vi "Main.vi"(8 "Error In":errorcluster) -> (0 "Error Out":errorcluster)   [LabVIEW 2017, in "File IO.lvlib"]
uses:
  File IO.lvlib
  Controls/Params.ctl
  Controls/Commands [enum].ctl
  System Control/CTLs/Params.ctl
  DAQ/Controls/Params.ctl
  DAQ/Controls/DAQ Config.ctl
  DAQ/Controls/DAQ Indicators.ctl
  System Control/CTLs/Test Type.ctl
  Shutter Module/Controls/Params.ctl
  Monochromator/Controls/VISA parameters.ctl
  Monochromator/Controls/Params.ctl
  Monochromator/Controls/Type.ctl
  Monochromator/Controls/GratingValues.ctl
  Monochromator/Controls/Grating.ctl
  Monochromator/PTI/Controls/Params.ctl
  Monochromator/Custom Oriel drivers/Controls/Params.ctl
  C:/Project Work/icl-optical-software-rewrite/Optical Software Code Simplified/Modules/Monochromator/Cornerstone.dll
  Monochromator/Cornerstone.dll
  System Control/CTLs/Test params.ctl
  System Control/CTLs/Test Controls.ctl
  System Control/CTLs/Test indicators.ctl
  Scope/Controls/Params.ctl
  Scope/Controls/Models.ctl
  Scope/Controls/TPC.ctl
  Scope/Controls/Channels.ctl
  Trigger/Controls/Params.ctl
  Trigger/Controls/Mode.ctl
  Trigger/Controls/Trigger channels.ctl
  Scope/Controls/Acquisition type.ctl
  Scope/Controls/Record length.ctl
  Scope/Controls/Data.ctl
  Scope/Controls/Channel data.ctl
  Colour Wheel/Controls/Params.ctl
  Events/Controls/Action Refs [enum].ctl
  Controls/Config Cluster.ctl
  <userlib>/_OpenG.lib/file/file.llb/Valid Path - Traditional__ogtk.vi
  <vilib>/Utility/error.llb/Error Cluster From Error Code.vi
  <vilib>/ErrorRing/Error Ring.xnode
  System Control/Main controller.lvlib
  Events/Events.lvlib
  <vilib>/Utility/config.llb/NI_LVConfig.lvlib
  DAQ/DAQ.lvlib
  Serial comms/Serial comms.lvlib
  Shutter Module/Shutter.lvlib
  Monochromator/Monochromator.lvlib
  Monochromator/PTI/PTI.lvlib
  Monochromator/Custom Oriel drivers/Oriel (custom drivers).lvlib
  Scope/Scope.lvlib
  Trigger/Trigger.lvlib
  Colour Wheel/Colour Wheel.lvlib
  Processing/Processing.lvlib
panel:
  in  "Config":T1={"DAQ"={"Data"={"Live"={"t0"=timestamp(0 s since 1904-01-01), "dt"=1.0, "Y"=[]}, "Accumulated"={"t0"=timestamp(0 s since 1904-01-01), "dt"=1.0, "Y"=[]}, "Averaged"={"t0"=timestamp(0 s since 1904-01-01), "dt"=1.0, "Y"=[]}, "data array"=[], "live time array"=[], "Live (decimated)"={"t0"=timestamp(0 s since 1904-01-01), "dt"=1.0, "Y"=[]}}, "Config"={"Input Config"=10106, "Card"=enum."USB-6211", "100% Reflectance Standard (V)"=1.0, "Input Channel"="Dev2/ai0", "Average number of points"=50.0, "Trigger Level (V)"=0.4, "Rate (Hz)"=250000, "End Time (s)"=1.0}, "Indicators"={"Final number of points"=0.0, "Number of samples"=0.0, "dt"=0.0, "Shots"=1, "Shot counter"=0, "Test counter"=0, "Background level (V)"=0.0, "DAQ task"="", "timestamp of data"=timestamp(0 s since 1904-01-01), "Test Type"=enum."A-Test"}}, "Shutter"={"Open command string"="", "VISA"={"Timeout (ms)"=0, "Resource Name"="", "Baud Rate"=0, "Data Bits"=0, "Parity"=0, "Stop Bits"=0, "Flow Control"=0}}, "Monochromator"={"Type"=enum."Oriel", "Wavelength (nm)"=0.0, "Grating, gr/mm"=enum."2400", "Grating mode"=enum."Unknown", "Spectrum mode"={"Spectrum mode?"=FALSE, "Start wavelength (nm)"=0.0, "End wavelength (nm)"=0.0, "Wavelength step (nm)"=0.0, "Wavelength array"=[], "array index"=0}, "PTI"={"Delay before read (ms)"=0, "Mono 1"={"Timeout (ms)"=0, "Resource Name"="", "Baud Rate"=0, "Data Bits"=0, "Parity"=0, "Stop Bits"=0, "Flow Control"=0}, "Mono 2"={"Timeout (ms)"=0, "Resource Name"="", "Baud Rate"=0, "Data Bits"=0, "Parity"=0, "Stop Bits"=0, "Flow Control"=0}, "Two PTI Monochromators?"=FALSE}, "Oriel (custom)"={"reference"=refnum}, "Force wavelength confirmation (PTI)?"=FALSE}, "Test"={"Config"={"Amplification Factor"=0.0, "100% Reflectance Standard"=0.0, "Calculation Method"=enum."Reflectance", "Option to discard new data?"=FALSE, "Mode"=enum."Spectrum", "Number of Averages"=0, "B Test?"=FALSE}, "Indicators"={"DAQ Background Level (V)"=0.0, "A-Test Counter"=0, "B-Test Counter"=0, "Type"=enum."A-Test", "Scope Background Level (Amps)"=2.0, "TAS only?"=FALSE}}, "Scope"={"Config"={"VISA Resource"="USB0::0x0699::0x039D::C010764::INSTR", "Model"=enum."DPO 2012B", "Timebase"=0.0004, "Timeout (ms)"=60000, "TAS"={"Vertical Range (V)"=2.0, "Vertical Offset (0.0 divs)"=0.0, "Bandwidth"=0, "Probe Attenuation (10.0)"=1.0, "Vertical Coupling"=1, "Impedance"=0, "Multiplication factor"=1.0, "Channel"=enum."Channel 1"}, "TPC"={"Vertical Range (V)"=2.0, "Vertical Offset (0.0 divs)"=0.0, "Bandwidth"=0, "Probe Attenuation (10.0)"=1.0, "Vertical Coupling"=1, "Impedance"=0, "Multiplication factor"=1.0, "Channel"=enum."None"}, "Trigger"={"Mode"=enum."Laser (TAS)", "Source "=enum."Aux", "PIA"={"Test LEDs"=FALSE, "LED line"="", "LED off (s)"=0.0, "LED on (s)"=0.0}, "Threshold (V)"=0.8}}, "Indicators"={"Setup"={"Final number of points"=0.0, "Pretrigger points"=0.0, "Number of readouts"=0, "Model"={"Acquisition Type"=4, "Record length (points)"=1000, "Averages on scope"=4, "Average number of points"=10.0}}, "Timestamp of Data"=timestamp(0 s since 1904-01-01)}, "Data"={"TPC"={"Live data"={"t0"=timestamp(0 s since 1904-01-01), "dt"=1.0, "Y"=[]}, "Averaged data"={"t0"=timestamp(0 s since 1904-01-01), "dt"=1.0, "Y"=[]}, "Accumulated data"={"t0"=timestamp(0 s since 1904-01-01), "dt"=1.0, "Y"=[]}, "Final data"={"t0"=timestamp(0 s since 1904-01-01), "dt"=1.0, "Y"=[]}}, "TAS"={"Live data"={"t0"=timestamp(0 s since 1904-01-01), "dt"=1.0, "Y"=[]}, "Averaged data"={"t0"=timestamp(0 s since 1904-01-01), "dt"=1.0, "Y"=[]}, "Accumulated data"={"t0"=timestamp(0 s since 1904-01-01), "dt"=1.0, "Y"=[]}, "Final data"={"t0"=timestamp(0 s since 1904-01-01), "dt"=1.0, "Y"=[]}}, "Time arrays"={"Time array (decimated)"=[], "waveform"={"t0"=timestamp(0 s since 1904-01-01), "dt"=1.0, "Y"=[]}}}, "Test"={"Config"={"Amplification Factor"=0.0, "100% Reflectance Standard"=0.0, "Calculation Method"=enum."Reflectance", "Option to discard new data?"=FALSE, "Mode"=enum."Spectrum", "Number of Averages"=100, "B Test?"=FALSE}, "Indicators"={"DAQ Background Level (V)"=2.0, "A-Test Counter"=2, "B-Test Counter"=2, "Type"=enum."A-Test", "Scope Background Level (Amps)"=2.0, "TAS only?"=FALSE}}}, "Colour wheel"={"Reference"=0, "Colour Wheel Wavelengths"=[], "Waveform Index"=0, "COM Port"="", "Enabled?"=FALSE}, "File IO"={"Output Folder"=path "C:/Users/Abigail/Documents/Imperial Optical software/Optical Software Code Simplified/Output", "Error file"=path "C:/Users/Abigail/Documents/Imperial Optical software/Optical Software Code Simplified/Error Log.txt", "Config file"=path "C:/Users/Abigail/Documents/Imperial Optical software/Optical Software Code Simplified/Config.ini", "File prefix"="", "Waveform read"={"t0"=timestamp(0 s since 1904-01-01), "dt"=1.0, "Y"=[]}}} {"Scope"."Test"."Config"."Number of Averages" min=0; "Scope"."Indicators"."Setup"."Model"."Record length (points)" items=["1000"=1, "10,000"=10, "100,000"=100, "1,000,000"=1000, "5,000,000"=5000, "10,000,000"=10000]; "Scope"."Indicators"."Setup"."Model"."Acquisition Type" items=["Sample", "Peak Detect", "Hi Res", "Envelope", "Average"]; "Scope"."Config"."Trigger"."Threshold (V)" format="%#_3f"; "Scope"."Config"."TPC"."Impedance" items=["1M", "75", "50"]; "Scope"."Config"."TPC"."Vertical Coupling" items=["AC", "DC", "Ground"]; "Scope"."Config"."TPC"."Bandwidth" items=["FULL", "250 MHz", "150 MHz", "20 MHz"]; "Scope"."Config"."TAS"."Impedance" items=["1M", "75", "50"]; "Scope"."Config"."TAS"."Vertical Coupling" items=["AC", "DC", "Ground"]; "Scope"."Config"."TAS"."Bandwidth" items=["FULL", "250 MHz", "150 MHz", "20 MHz"]; "Scope"."Config"."Timebase" format="%^#_3e"; "Test"."Config"."Number of Averages" min=0; "Monochromator"."PTI"."Mono 2"."Flow Control" items=["1.0"=10, "1.5"=15, "2.0"=20]; "Monochromator"."PTI"."Mono 2"."Stop Bits" items=["None", "Odd", "Even", "Mark", "Space"]; "Monochromator"."PTI"."Mono 2"."Parity" items=["None", "Odd", "Even", "Mark", "Space"]; "Monochromator"."PTI"."Mono 1"."Flow Control" items=["1.0"=10, "1.5"=15, "2.0"=20]; "Monochromator"."PTI"."Mono 1"."Stop Bits" items=["None", "Odd", "Even", "Mark", "Space"]; "Monochromator"."PTI"."Mono 1"."Parity" items=["None", "Odd", "Even", "Mark", "Space"]; "Shutter"."VISA"."Flow Control" items=["None"=0, "XON/XOFF"=1, "RTS/CTS"=2, "DTR/DSR"=4]; "Shutter"."VISA"."Stop Bits" items=["1.0"=10, "1.5"=15, "2.0"=20]; "Shutter"."VISA"."Parity" items=["None", "Odd", "Even", "Mark", "Space"]; "DAQ"."Config"."Input Config" items=["default"=-1, "RSE"=10083, "NRSE"=10078, "Differential"=10106, "Pseudodifferential"=12529]}
  in  "State":T30
  in  "Stop Button":bool
  in  "Config":T29={"Output Folder"=path "C:/Users/Abigail/Documents/Imperial Optical software/Optical Software Code Simplified/Output", "Error file"=path "Error Log.txt", "Config file"=path "Config.ini", "File prefix"="600nm", "Waveform read"={"t0"=timestamp(0 s since 1904-01-01), "dt"=1.0, "Y"=[]}}
  out "Test":bool=TRUE
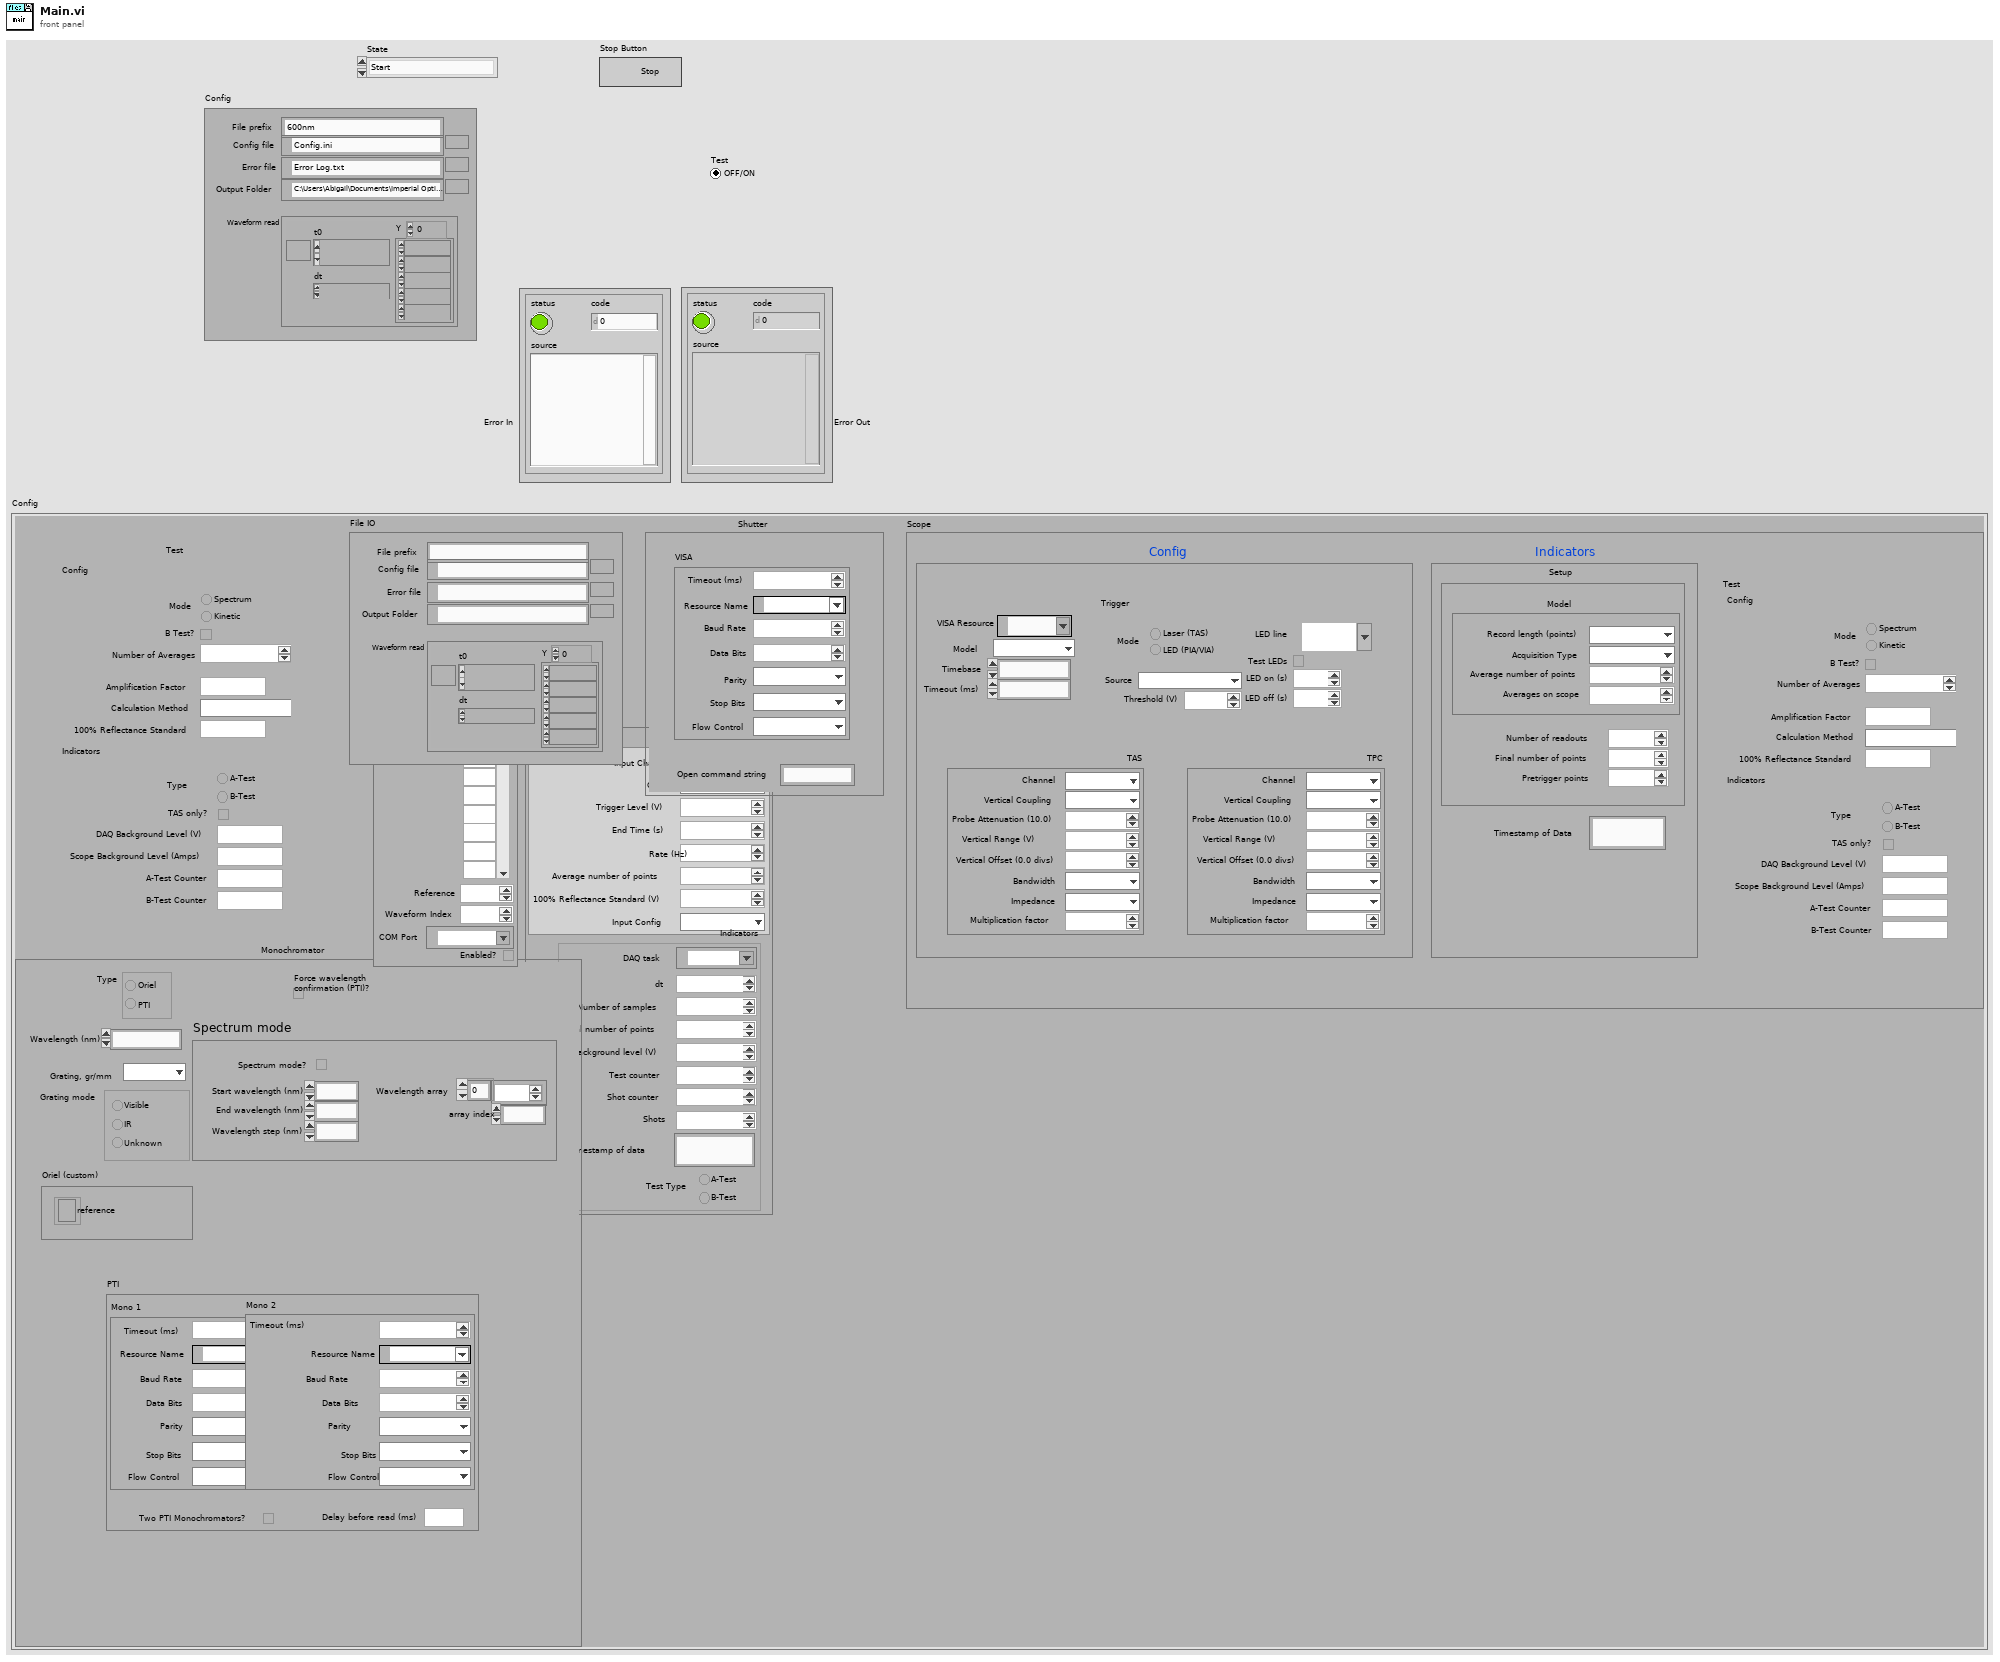
[diagram p1: front panel]
types:
  T1 = typedef "Main controller.lvlib/Params.ctl" = cluster{"DAQ":T2, "Shutter":T6, "Monochromator":T8, "Test":T14, "Scope":T17, "Colour wheel":T28, "File IO":T29}
  T2 = typedef "DAQ.lvlib/Params.ctl" = cluster{"Data":cluster{"Live":waveform(dbl), "Accumulated":waveform(dbl), "Averaged":waveform(dbl), "data array":dbl[], "live time array":dbl[], "Live (decimated)":waveform(dbl)}, "Config":T3, "Indicators":T4}
  T3 = typedef "DAQ.lvlib/DAQ Config.ctl" = cluster{"Input Config":i32, "Card":enum16{"USB-6211", "USB-6251", "USB-6361"}, "100% Reflectance Standard (V)":dbl, "Input Channel":tag, "Average number of points":dbl, "Trigger Level (V)":dbl, "Rate (Hz)":i32, "End Time (s)":dbl}
  T4 = typedef "DAQ.lvlib/DAQ Indicators.ctl" = cluster{"Final number of points":dbl, "Number of samples":dbl, "dt":dbl, "Shots":i32, "Shot counter":i32, "Test counter":i32, "Background level (V)":dbl, "DAQ task":refnum<k21>, "timestamp of data":timestamp, "Test Type":T5}
  T5 = typedef "Main controller.lvlib/Test Type.ctl" = enum32{"A-Test", "B-Test"}
  T6 = typedef "Shutter.lvlib/Params.ctl" = cluster{"Open command string":string, "VISA":T7}
  T7 = typedef "Serial comms.lvlib/VISA parameters.ctl" = cluster{"Timeout (ms)":u32, "Resource Name":refnum<visa-resource-name>, "Baud Rate":u32, "Data Bits":u16, "Parity":u16, "Stop Bits":u16, "Flow Control":u16}
  T8 = typedef "Monochromator.lvlib/Params.ctl" = cluster{"Type":T9, "Wavelength (nm)":dbl, "Grating, gr/mm":T10, "Grating mode":T11, "Spectrum mode":cluster{"Spectrum mode?":bool, "Start wavelength (nm)":dbl, "End wavelength (nm)":dbl, "Wavelength step (nm)":dbl, "Wavelength array":dbl[], "array index":u32}, "PTI":T12, "Oriel (custom)":T13, "Force wavelength confirmation (PTI)?":bool}
  T9 = typedef "Monochromator.lvlib/Type.ctl" = enum32{"Oriel", "PTI"}
  T10 = typedef "Monochromator.lvlib/GratingValues.ctl" = enum16{"2400", "1800", "1200", "600", "300", "150"}
  T11 = typedef "Monochromator.lvlib/Grating.ctl" = enum32{"Unknown", "Visible", "IR"}
  T12 = typedef "Monochromator.lvlib/PTI.lvlib/Params.ctl" = cluster{"Delay before read (ms)":u32, "Mono 1":T7, "Mono 2":T7, "Two PTI Monochromators?":bool}
  T13 = typedef "Monochromator.lvlib/Oriel (custom drivers).lvlib/Params.ctl" = cluster{"reference":refnum<k24>}
  T14 = typedef "Main controller.lvlib/Test params.ctl" = cluster{"Config":T15, "Indicators":T16}
  T15 = typedef "Main controller.lvlib/Test Controls.ctl" = cluster{"Amplification Factor":dbl, "100% Reflectance Standard":dbl, "Calculation Method":enum16{"Reflectance", "Transmission", "Kubelka-Munk"}, "Option to discard new data?":bool, "Mode":enum32{"Spectrum", "Kinetic"}, "Number of Averages":i32, "B Test?":bool}
  T16 = typedef "Main controller.lvlib/Test indicators.ctl" = cluster{"DAQ Background Level (V)":dbl, "A-Test Counter":i32, "B-Test Counter":i32, "Type":T5, "Scope Background Level (Amps)":dbl, "TAS only?":bool}
  T17 = typedef "Scope.lvlib/Params.ctl" = cluster{"Config":cluster{"VISA Resource":refnum<visa-resource-name>, "Model":T18, "Timebase":dbl, "Timeout (ms)":u32, "TAS":T19, "TPC":T19, "Trigger":T21}, "Indicators":cluster{"Setup":cluster{"Final number of points":dbl, "Pretrigger points":dbl, "Number of readouts":i32, "Model":cluster{"Acquisition Type":T24, "Record length (points)":T25, "Averages on scope":i32, "Average number of points":dbl}}, "Timestamp of Data":timestamp}, "Data":T26, "Test":T14}
  T18 = typedef "Scope.lvlib/Models.ctl" = enum16{"DPO 3012", "DPO 2012B", "TDS 3012C"}
  T19 = typedef "Scope.lvlib/TPC.ctl" = cluster{"Vertical Range (V)":dbl, "Vertical Offset (0.0 divs)":dbl, "Bandwidth":i32, "Probe Attenuation (10.0)":dbl, "Vertical Coupling":u16, "Impedance":u16, "Multiplication factor":dbl, "Channel":T20}
  T20 = typedef "Scope.lvlib/Channels.ctl" = enum16{"Channel 1", "Channel 2", "Channel 3", "Channel 4", "Math", "Reference A", "Reference B", "Reference C", "Reference D", "B1", "B2", "None"}
  T21 = typedef "Scope.lvlib/Trigger.lvlib/Params.ctl" = cluster{"Mode":T22, "Source ":T23, "PIA":cluster{"Test LEDs":bool, "LED line":tag, "LED off (s)":dbl, "LED on (s)":dbl}, "Threshold (V)":dbl}
  T22 = typedef "Scope.lvlib/Trigger.lvlib/Mode.ctl" = enum32{"Laser (TAS)", "LED (PIA/VIA)"}
  T23 = typedef "Scope.lvlib/Trigger.lvlib/Trigger channels.ctl" = enum16{"Channel 1", "Channel 2", "Channel 3", "Channel 4", "AC Line", "Aux", "Digital Channel 0", "Digital Channel 1", "Digital Channel 2", "Digital Channel 3", "Digital Channel 4", "Digital Channel 5", "Digital Channel 6", "Digital Channel 7", "Digital Channel 8", "Digital Channel 9", "Digital Channel 10", "Digital Channel 11", "Digital Channel 12", "Digital Channel 13", "Digital Channel 14", "Digital Channel 15", "RF"}
  T24 = typedef "Scope.lvlib/Acquisition type.ctl" = u16
  T25 = typedef "Scope.lvlib/Record length.ctl" = u32
  T26 = typedef "Scope.lvlib/Data.ctl" = cluster{"TPC":T27, "TAS":T27, "Time arrays":cluster{"Time array (decimated)":dbl[], "waveform":waveform(dbl)}}
  T27 = typedef "Scope.lvlib/Channel data.ctl" = cluster{"Live data":waveform(dbl), "Averaged data":waveform(dbl), "Accumulated data":waveform(dbl), "Final data":waveform(dbl)}
  T28 = typedef "Colour Wheel.lvlib/Params.ctl" = cluster{"Reference":i32, "Colour Wheel Wavelengths":dbl[], "Waveform Index":i32, "COM Port":refnum<visa-resource-name>, "Enabled?":bool}
  T29 = typedef "File IO.lvlib/Params.ctl" = cluster{"Output Folder":path, "Error file":path, "Config file":path, "File prefix":string, "Waveform read":waveform(dbl)}
  T30 = typedef "File IO.lvlib/Commands [enum].ctl" = enum16{"Start", "Stop", "Read waveform", "Write waveform", "Delete waveform", "Log error", "Write config", "Read config", "Save parameters", "Send waveform to processing", "Update file prefix"}
  T31 = enum32{"Bad", "Idle", "Run top level", "Running"}
  T32 = typedef "Events.lvlib/Action Refs [enum].ctl" = enum16{"Init", "Ref", "Kill"}
  T33 = typedef "Events.lvlib/Refs [cluster].ctl" = cluster{"Exit":refnum<user-event>, "Controller":refnum<user-event>, "System Error":refnum<user-event>, "UI":refnum<user-event>, "Example Module":refnum<user-event>, "Shutter":refnum<user-event>, "Monochromator":refnum<user-event>, "DAQ":refnum<user-event>, "Scope":refnum<user-event>, "Processing":refnum<user-event>, "File IO":refnum<user-event>, "Colour wheel":refnum<user-event>}
  T34 = enum16{"open", "replace", "create", "open or create", "replace or create", "replace or create with confirmation"}
  T35 = cluster{"Waveform Data":dbl[][], "Waveform Name":string}
  T36 = cluster{"Debug Waveform Read":dbl[][], "Waveform name":string}
  T37 = typedef "File IO.lvlib/Config Cluster.ctl" = cluster{"Test.Config":T15, "File IO":T29, "DAQ.Config":T3, "Monochromator":T8, "Scope.Config":cluster{"VISA Resource":refnum<visa-resource-name>, "Model":T18, "Timebase":dbl, "Timeout (ms)":u32, "TAS":T19, "TPC":T19, "Trigger":T21}, "Colour Wheel":T28, "Shutter":T6, "Scope.Setup.Model":cluster{"Acquisition Type":T24, "Record length (points)":T25, "Averages on scope":i32, "Average number of points":dbl}}
  T38 = typedef "NI_LVConfig.lvlib/Config Data RefNum.ctl" = refnum<k1>
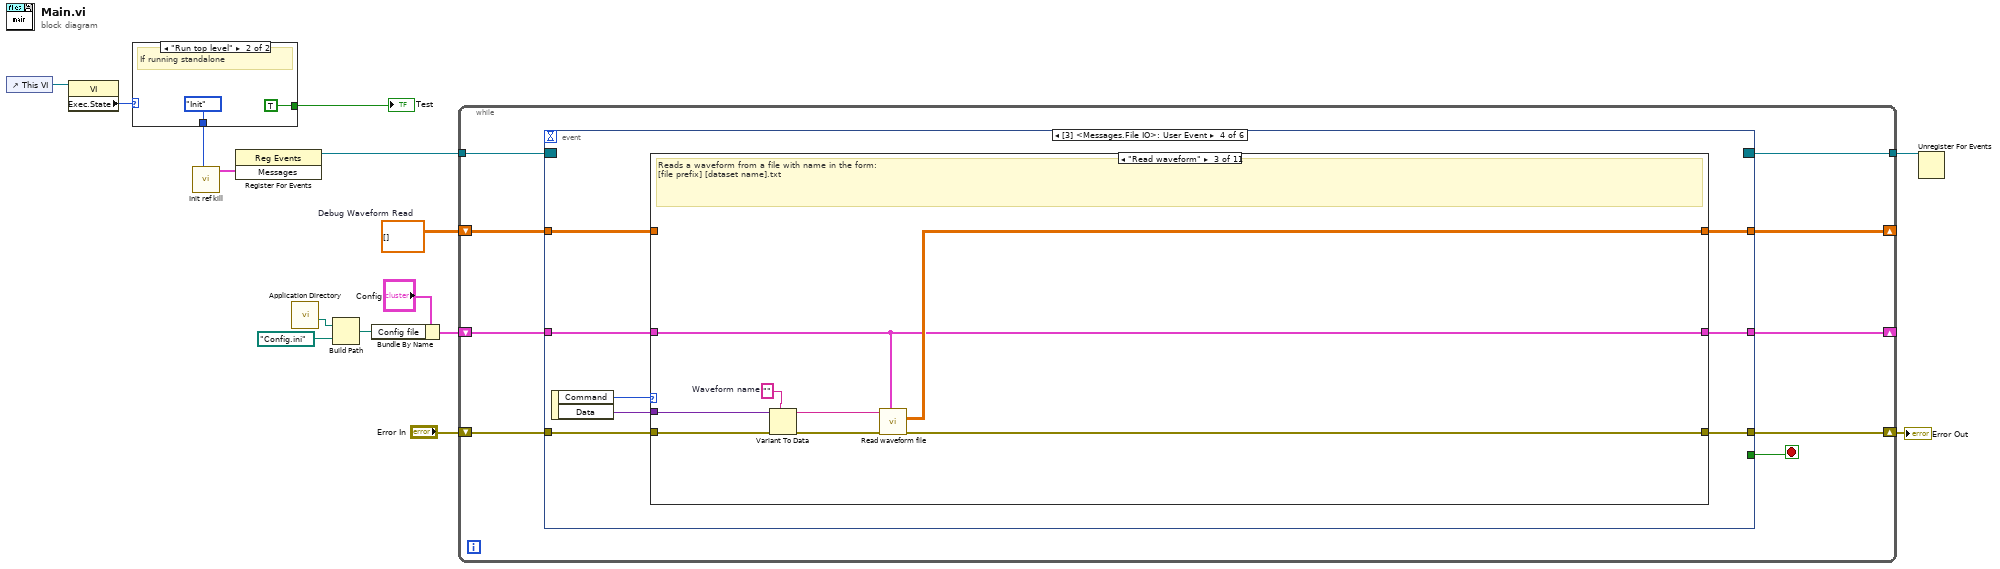
[diagram p0: block diagram]
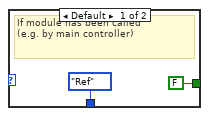
[diagram p2: hidden frame]
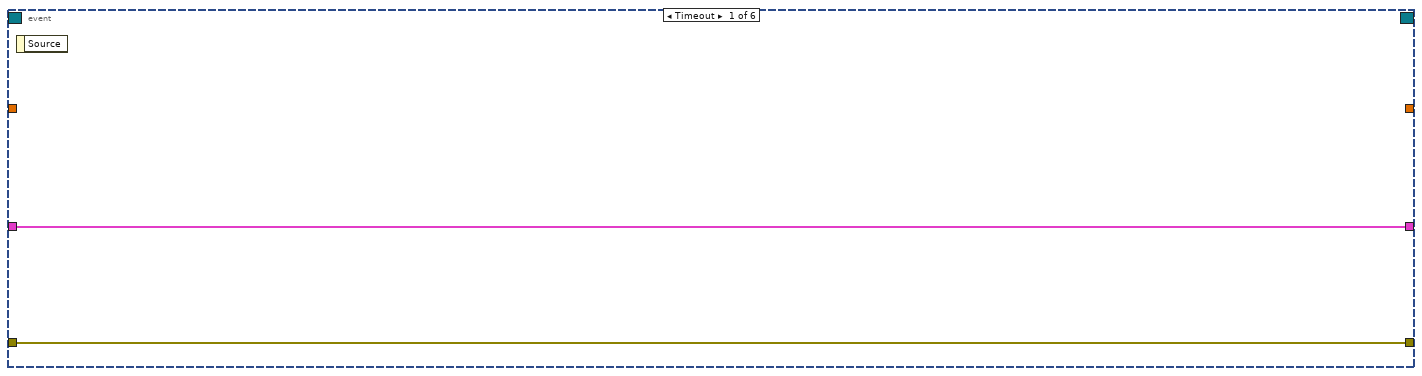
[diagram p3: hidden frame]
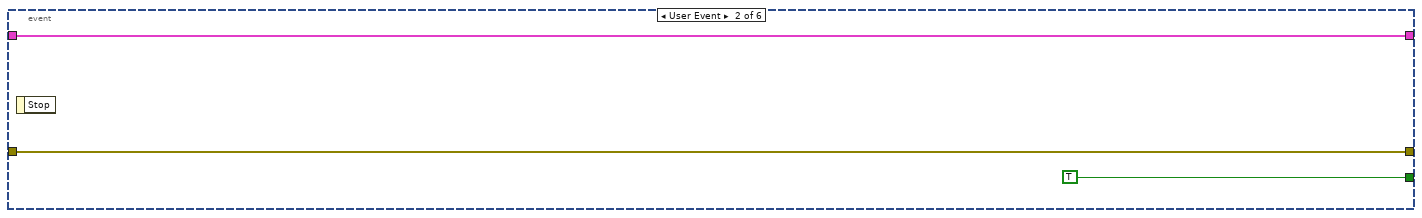
[diagram p4: hidden frame]
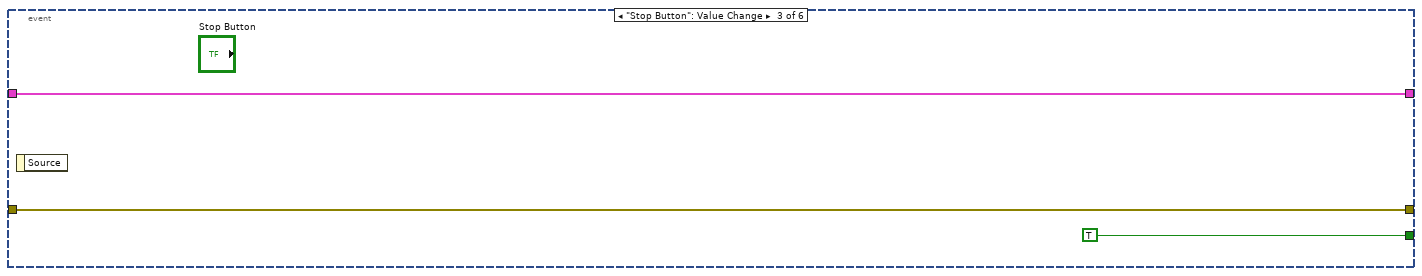
[diagram p5: hidden frame]
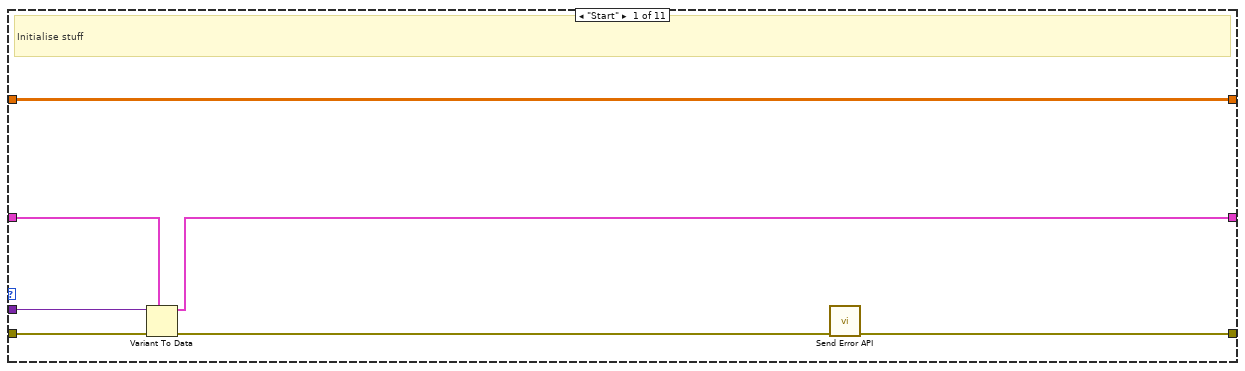
[diagram p6: hidden frame]
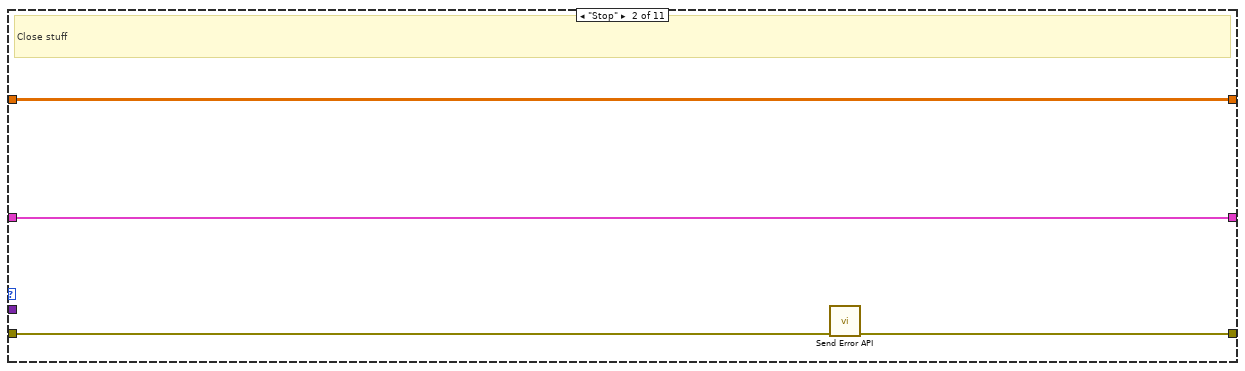
[diagram p7: hidden frame]
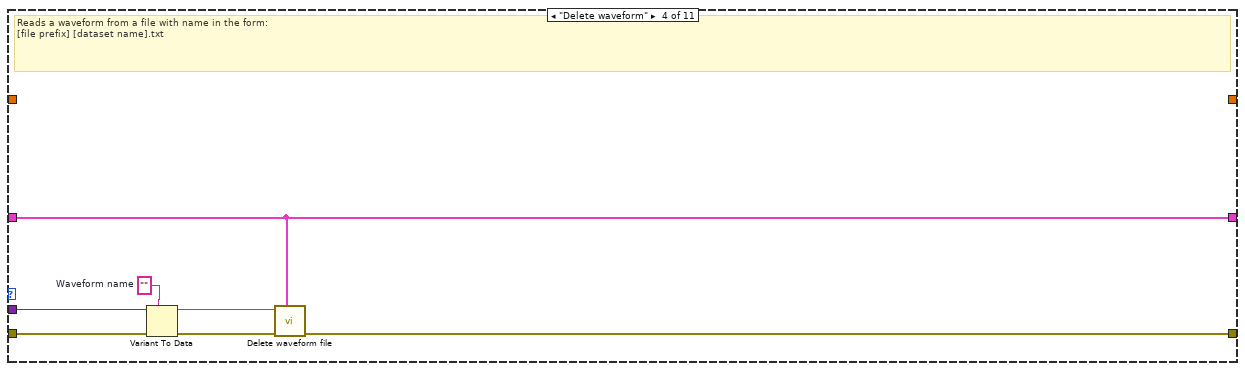
[diagram p8: hidden frame]
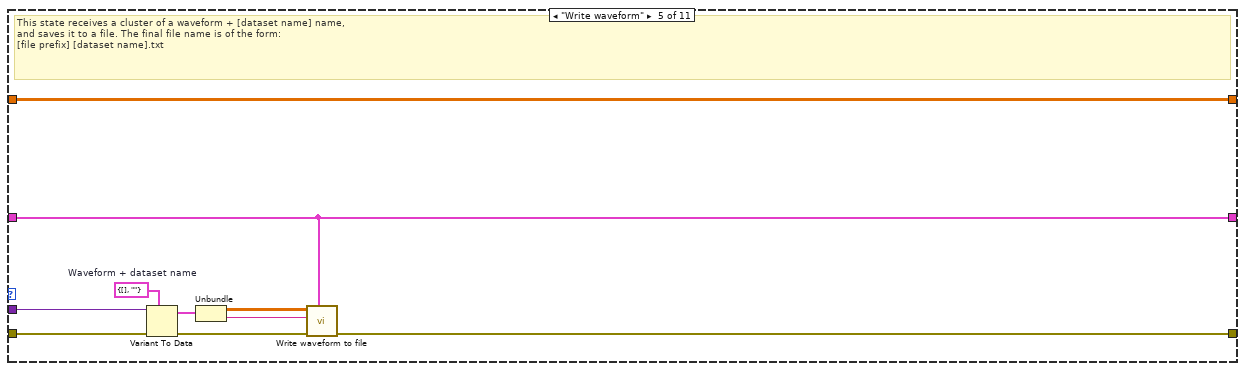
[diagram p9: hidden frame]
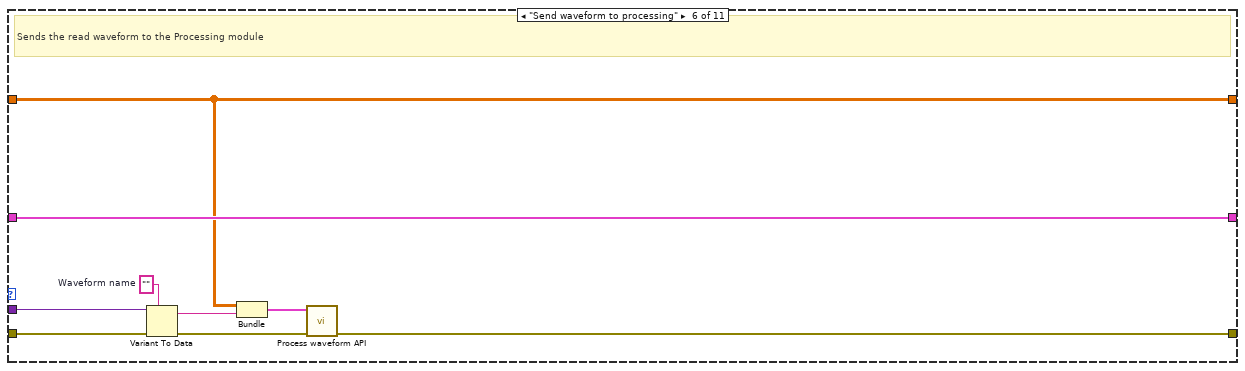
[diagram p10: hidden frame]
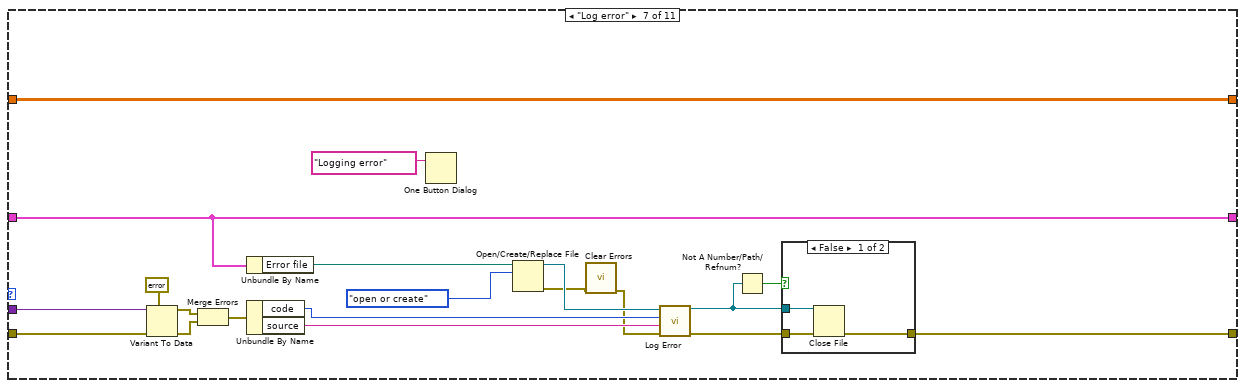
[diagram p11: hidden frame]
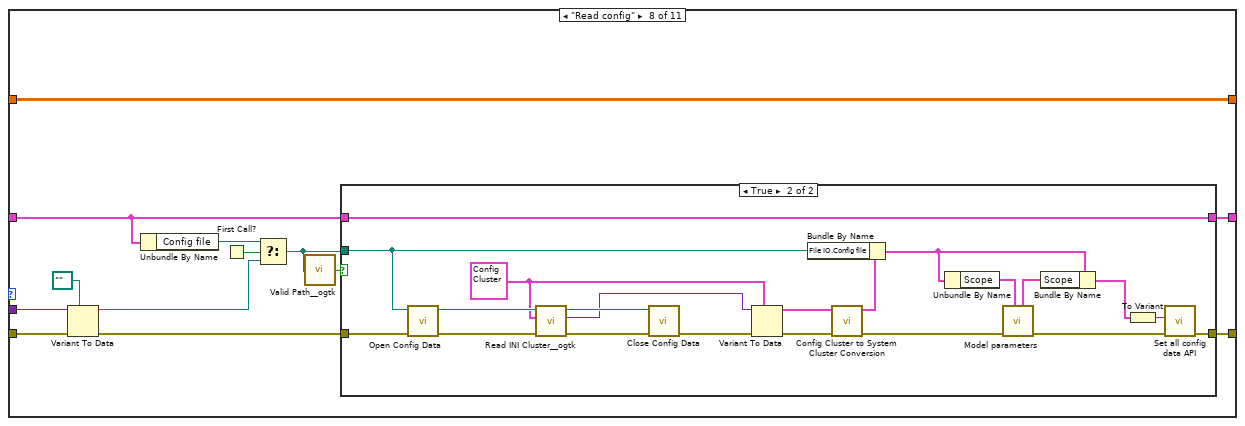
[diagram p13: hidden frame]
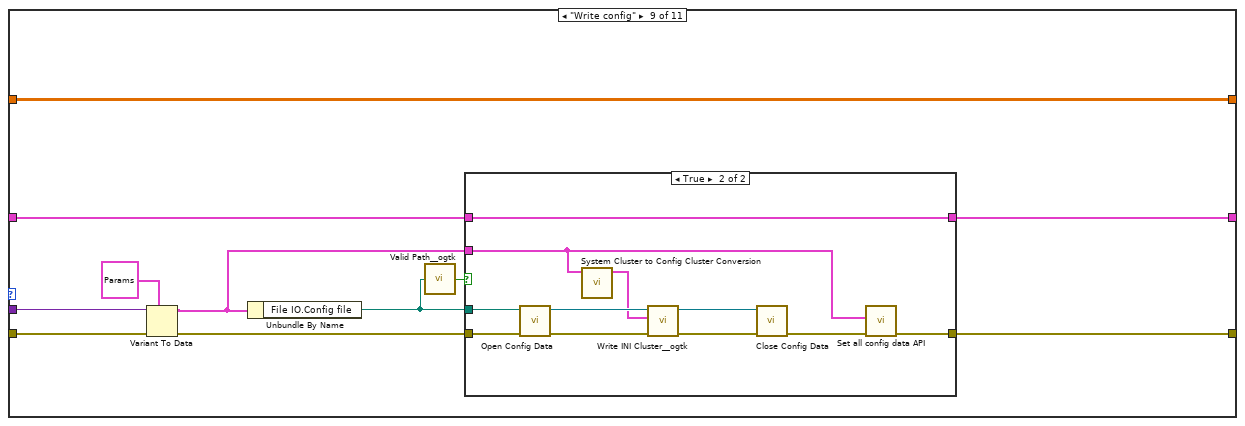
[diagram p15: hidden frame]
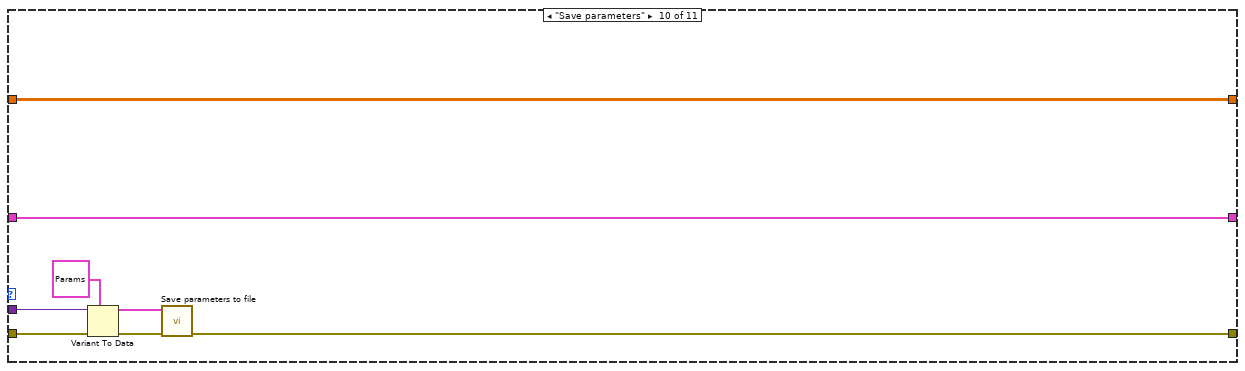
[diagram p17: hidden frame]
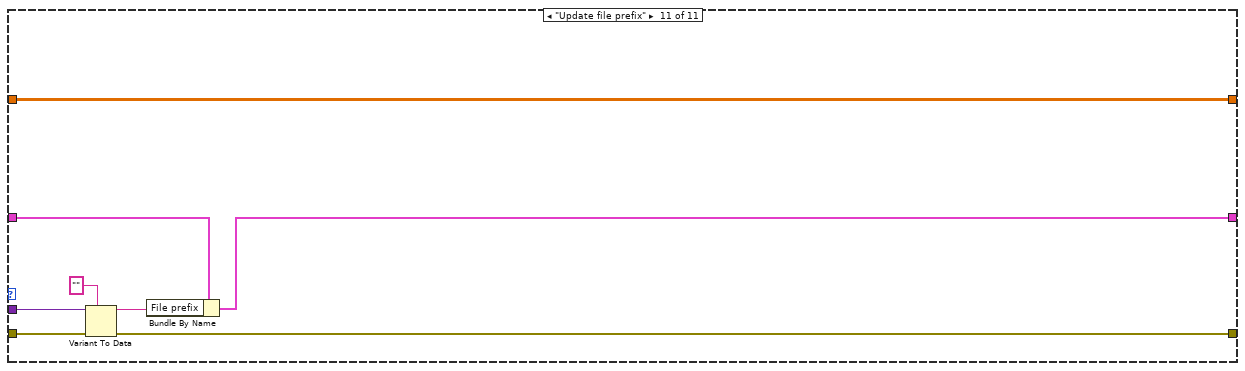
[diagram p18: hidden frame]
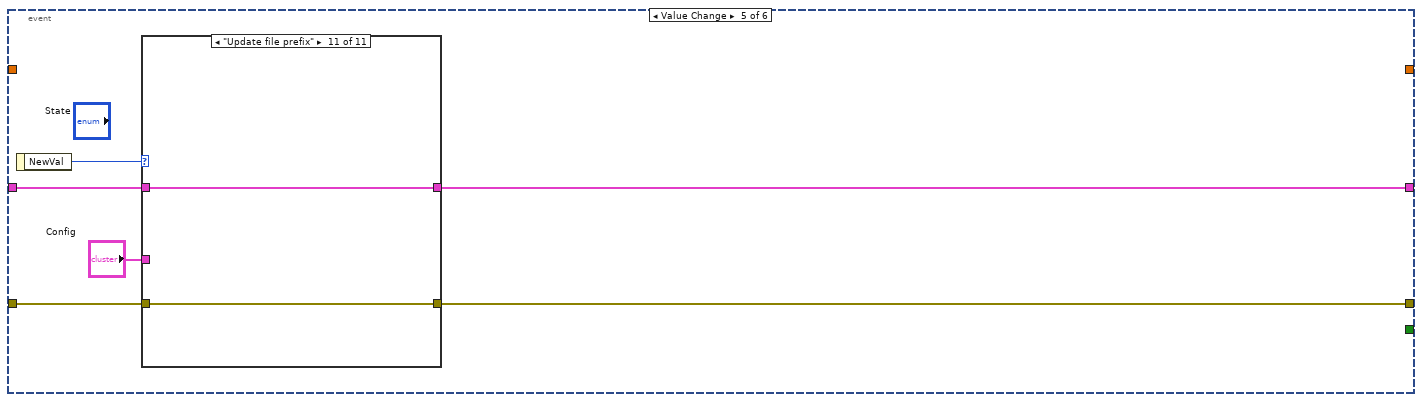
[diagram p19: hidden frame]
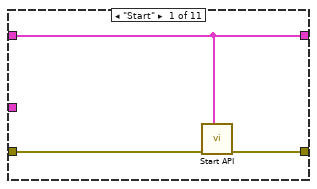
[diagram p20: hidden frame]
diagram:
  w1 = dbl[][] []  # Debug Waveform Read
  n1 = control-ref of="This VI"() -> (w10:refnum<vi>)
  n2 = property class="VI"(reference=w10) -> ("Exec.State"=w9:T31)  [unwired: 1 in, 2 out]
  n3 = case shown="\"Run top level\"" w9 {
    tunnel: [Action_Refs_[enum]."Ref" ("Action") Action_Refs_[enum]."Init" ("Action")] -> w7
    tunnel: [FALSE TRUE] -> w8
    frame Default {
      # "If module has been called\n(e.g. by main controller)"
    }
    frame "Run top level" {
      # "If running standalone"
    }
  }
  "Test" <- w8
  n4 = call "Init ref kill.vi"("Action"=w7) -> ("Messages"=w15:T33)  [unwired: 9 in, 1 out]
  n5 = register-events(w15) -> (reference out=w14:refnum<event-registration>)  [unwired: 2 in, 1 out]
  n6 = call <vilib>:"Application Directory.vi"() -> ("Application Directory"=w4:path)
  n7 = Build Path(base path=w4, name or relative path=path "Config.ini" ("Error file")) -> (appended path=w5:path)
  n8 = Bundle By Name(cluster="Config", "Config file"=w5) -> (w2:T29)
  n9 = while {
    tunnel: w14 -> [w28]
    tunnel: [w26] -> w13
    shift-right: [w20] -> w11
    shift-left: "Error In" -> [w25]
    shift-right: [w23] -> _
    shift-left: w2 -> [w24]
    shift-right: [w22] -> _
    shift-left: w1 -> [w21]
    stop <- w27 stop-if-true
    n10 = event shown="[3] <Messages.File IO>: User Event" {
      selector: w28 -> [_ _ _ _ _ _]
      dyn-events: [_ _ _ _ _ _] -> w26
      timeout: _ -> [_ _ _ _ _ _]
      tunnel: [_ TRUE TRUE _ _ _] -> w27
      tunnel: w25 -> [w29 w31 w36 w42 w194 _]
      tunnel: [w29 w31 w36 w41 w195 w236] -> w20
      tunnel: w24 -> [w30 w32 w35 w40 w192 w238]
      tunnel: [w30 w32 w35 w39 w191 w238] -> w23
      tunnel: [_ _ _ w38 _ _] -> w22
      tunnel: w21 -> [_ _ _ w37 _ _]
      event Timeout {
        n11 = event-data() -> ()  [unwired: 1 in, 1 out]
      }
      event User Event {
        n12 = event-data() -> ()  [unwired: 1 in, 1 out]
      }
      event "Stop Button": Value Change {
        n13 = event-data() -> ()  [unwired: 1 in, 1 out]
      }
      event User Event {
        n14 = event-data() -> ("Command"=w44:T30, "Data"=w43:variant)  [unwired: 1 in]
        n15 = case shown="\"Read waveform\"" w44 {
          tunnel: w43 -> [w48 _ w62 w69 w77 w85 w98 w121 w158 w179 w188]
          tunnel: w42 -> [w50 w53 w63 w70 w79 w87 w96 w120 w156 w178 w187]
          tunnel: [w51 w54 w60 w67 w80 w88 w97 w126 w160 w175 w186] -> w41
          tunnel: w40 -> [w47 w55 w56 w64 w72 w89 w93 w123 w151 w181 w183]
          tunnel: [w46 w55 w56 w64 w72 w89 w93 w124 w153 w181 w182] -> w39
          tunnel: [w45 w52 w57 _ w71 w81 w90 w122 w152 w180 w189] -> w38
          tunnel: w37 -> [w45 w52 _ _ w71 w81 w90 w122 w152 w180 w189]
          frame "Start" {
            # "Initialise stuff"
            n16 = Variant To Data(error in=w50, type=w47, Variant=w48) -> (data=w46:T29, error out=w49:errorcluster)
            n17 = call "Send Error API.vi"("Error Cluster"=w49) -> ("Error Out"=w51:errorcluster)  [unwired: 10 in]
          }
          frame "Stop" {
            # "Close stuff"
            n18 = call "Send Error API.vi"("Error Cluster"=w53) -> ("Error Out"=w54:errorcluster)  [unwired: 10 in]
          }
          frame "Read waveform" {
            w58 = ""  # Waveform name
            # "Reads a waveform from a file with name in the form: \n[file prefix] [dataset name].txt"
            n19 = Variant To Data(error in=w63, type=w58, Variant=w62) -> (data=w59:string, error out=w61:errorcluster)
            n20 = call "Read waveform file.vi"("File IO parameters"=w56, "error in"=w61, "Dataset name"=w59) -> ("error out"=w60:errorcluster, "all rows"=w57:dbl[][])  [unwired: 6 in, 1 out]
          }
          frame "Delete waveform" {
            w65 = ""  # Waveform name
            # "Reads a waveform from a file with name in the form: \n[file prefix] [dataset name].txt"
            n21 = Variant To Data(error in=w70, type=w65, Variant=w69) -> (data=w66:string, error out=w68:errorcluster)
            n22 = call "Delete waveform file.vi"("File IO parameters"=w64, "error in"=w68, "Dataset name"=w66) -> ("error out"=w67:errorcluster)  [unwired: 8 in]
          }
          frame "Write waveform" {
            w75 = T35 {"Waveform Data"=[], "Waveform Name"=""}  # Waveform + dataset name
            # "This state receives a cluster of a waveform + [dataset name] name, \nand saves it to a file. The final file name is of the form: \n[file prefix] [dataset name].txt"
            n23 = Variant To Data(error in=w79, type=w75, Variant=w77) -> (data=w76:T35, error out=w78:errorcluster)
            n24 = Unbundle(w76) -> ("Waveform Data"=w74:dbl[][], "Waveform Name"=w73:string)
            n25 = call "Write waveform to file.vi"("File IO parameters"=w72, "error in"=w78, "Dataset name"=w73, "Data"=w74) -> ("error out"=w80:errorcluster)  [unwired: 7 in]
          }
          frame "Send waveform to processing" {
            w82 = ""  # Waveform name
            # "Sends the read waveform to the Processing module"
            n26 = Variant To Data(error in=w87, type=w82, Variant=w85) -> (data=w84:string, error out=w86:errorcluster)
            n27 = Bundle("Debug Waveform Read"=w81, "Waveform name"=w84) -> (w83:T36)  [unwired: 1 in]
            n28 = call "Process waveform API.vi"("Error In"=w86, "Waveform + name 2"=w83) -> ("Error Out"=w88:errorcluster)  [unwired: 9 in]
          }
          frame "Log error" {
            n29 = Variant To Data(error in=w96, type=errorcluster {"status"=FALSE, "code"=0, "source"=""} ("error out"), Variant=w98) -> (data=w107:errorcluster, error out=w108:errorcluster)
            n30 = Merge Errors(w107, w108) -> (w105:errorcluster)
            n31 = Unbundle By Name(w93) -> ("Error file"=w92:path)
            n32 = Unbundle By Name(w105) -> ("code"=w104:i32, "source"=w103:string)
            n33 = One Button Dialog(message="Logging error") -> ()  [unwired: 1 in, 1 out]
            n34 = Open/Create/Replace File(file path (use dialog)=w92, operation (0:open)=T34."open or create") -> (refnum out=w109:refnum<file>, error out=w95:errorcluster)  [unwired: 4 in, 1 out]
            n35 = call <vilib>:"Clear Errors.vi"("error in (no error)"=w95) -> ("error out"=w94:errorcluster)  [unwired: 5 in, 1 out]
            n36 = call "Log Error.vi"("error in"=w94, "Source"=w103, "Code"=w104, "Error Log Refnum In"=w109) -> ("error out"=w101:errorcluster, "Error Log Refnum Out"=w100:refnum<file>)  [unwired: 6 in]
            n37 = Not A Number/Path/Refnum?(number/path/refnum=w100) -> (NaN/Path/Refnum?=w102:bool)
            n38 = case shown="False" w102 {
              tunnel: [w112 w113] -> w97
              tunnel: w101 -> [w111 w113]
              tunnel: w100 -> [w110 _]
              frame False {
                n39 = Close File(refnum=w110, error in=w111) -> (error out=w112:errorcluster)  [unwired: 1 out]
              }
              frame True {
              }
            }
          }
          frame "Read config" {
            n40 = Variant To Data(error in=w120, type=path "" ("Config file"), Variant=w121) -> (data=w114:path, error out=w119:errorcluster)
            n41 = Unbundle By Name(w123) -> ("Config file"=w117:path)
            n42 = First Call?() -> (First Call?: T/F=w118:bool)
            n43 = Select(t=w117, s=w118, f=w114) -> (s? t:f=w116:path)
            n44 = call-poly <userlib>:"Valid Path__ogtk.vi"("path"=w116) -> ("valid"=w125:bool)
            n45 = case shown="True" w125 {
              tunnel: [w128 w149] -> w126
              tunnel: w119 -> [w128 w147]
              tunnel: w116 -> [_ w141]
              tunnel: [w127 w143] -> w124
              tunnel: w123 -> [w127 w143]
              frame False {
              }
              frame True {
                w135 = T37 {"Test.Config"={"Amplification Factor"=0.0, "100% Reflectance Standard"=0.0, "Calculation Method"=enum."Reflectance", "Option to discard new data?"=FALSE, "Mode"=enum."Kinetic", "Number of Averages"=0, "B Test?"=FALSE}, "File IO"={"Output Folder"=path "C:/Users/Abigail/Documents/Imperial Optical software/Optical Software Code Simplified/Output", "Error file"=path "Error Log.txt", "Config file"=path "Config.ini", "File prefix"="", "Waveform read"={"t0"=timestamp(0 s since 1904-01-01), "dt"=1.0, "Y"=[]}}, "DAQ.Config"={"Input Config"=10106, "Card"=enum."USB-6251", "100% Reflectance Standard (V)"=1.0, "Input Channel"="Dev1/ai0", "Average number of points"=10.0, "Trigger Level (V)"=0.2, "Rate (Hz)"=1250000, "End Time (s)"=10.0}, "Monochromator"={"Type"=enum."PTI", "Wavelength (nm)"=600.0, "Grating, gr/mm"=enum."1200", "Grating mode"=enum."Unknown", "Spectrum mode"={"Spectrum mode?"=FALSE, "Start wavelength (nm)"=0.0, "End wavelength (nm)"=0.0, "Wavelength step (nm)"=0.0, "Wavelength array"=[], "array index"=0}, "PTI"={"Delay before read (ms)"=50, "Mono 1"={"Timeout (ms)"=1000, "Resource Name"="COM1", "Baud Rate"=9600, "Data Bits"=8, "Parity"=0, "Stop Bits"=10, "Flow Control"=0}, "Mono 2"={"Timeout (ms)"=1000, "Resource Name"="COM1", "Baud Rate"=9600, "Data Bits"=8, "Parity"=0, "Stop Bits"=10, "Flow Control"=0}, "Two PTI Monochromators?"=FALSE}, "Oriel (custom)"={"reference"=refnum}, "Force wavelength confirmation (PTI)?"=FALSE}, "Scope.Config"={"VISA Resource"="", "Model"=enum."DPO 3012", "Timebase"=0.0, "Timeout (ms)"=0, "TAS"={"Vertical Range (V)"=0.0, "Vertical Offset (0.0 divs)"=0.0, "Bandwidth"=0, "Probe Attenuation (10.0)"=0.0, "Vertical Coupling"=0, "Impedance"=0, "Multiplication factor"=0.0, "Channel"=enum."Channel 1"}, "TPC"={"Vertical Range (V)"=0.0, "Vertical Offset (0.0 divs)"=0.0, "Bandwidth"=0, "Probe Attenuation (10.0)"=0.0, "Vertical Coupling"=0, "Impedance"=0, "Multiplication factor"=0.0, "Channel"=enum."Channel 1"}, "Trigger"={"Mode"=enum."Laser (TAS)", "Source "=enum."Channel 1", "PIA"={"Test LEDs"=FALSE, "LED line"="", "LED off (s)"=0.0, "LED on (s)"=0.0}, "Threshold (V)"=0.0}}, "Colour Wheel"={"Reference"=0, "Colour Wheel Wavelengths"=[], "Waveform Index"=0, "COM Port"="", "Enabled?"=FALSE}, "Shutter"={"Open command string"="+100\\s10\\n", "VISA"={"Timeout (ms)"=1000, "Resource Name"="", "Baud Rate"=9600, "Data Bits"=9600, "Parity"=8, "Stop Bits"=0, "Flow Control"=10}}, "Scope.Setup.Model"={"Acquisition Type"=0, "Record length (points)"=0, "Averages on scope"=0, "Average number of points"=0.0}} ("Config Cluster")
                n46 = call <vilib>:"Open Config Data.vi"("error in (no error)"=w147, "configuration file path"=w141) -> ("error out"=w146:errorcluster, "refnum"=w148:T38)  [unwired: 7 in, 1 out]
                n47 = call <userlib>:"Read INI Cluster__ogtk.vi"("error in (no error)"=w146, "INI Fomatted Cluster Type"=w135, "refnum"=w148) -> ("error out"=w145:errorcluster, "INI Fomatted Cluster"=w142:variant, "dup refnum"=w144:T38)  [unwired: 4 in, 2 out]
                n48 = call <vilib>:"Close Config Data.vi"("error in (no error)"=w145, "refnum"=w144) -> ("error out"=w139:errorcluster)  [unwired: 8 in, 1 out]
                n49 = Variant To Data(error in=w139, type=w135, Variant=w142) -> (data=w138:T37, error out=w136:errorcluster)
                n50 = call "Config Cluster to System Cluster Conversion.vi"("error in (no error)"=w136, "Config Cluster"=w138) -> ("error out"=w132:errorcluster, "System Cluster"=w137:T1)  [unwired: 8 in]
                n51 = Bundle By Name(cluster=w137, "File IO.Config file"=w141) -> (w130:T1)
                n52 = Unbundle By Name(w130) -> ("Scope"=w134:T17)
                n53 = call "Model parameters.vi"("Scope"=w134, "error in"=w132) -> ("error out"=w131:errorcluster, "Scope out"=w133:T17)  [unwired: 8 in]
                n54 = Bundle By Name(cluster=w130, "Scope"=w133) -> (w129:T1)
                n55 = To Variant(anything=w129) -> (Variant=w140:variant)
                n56 = call "Set all config data API.vi"("Error In"=w131, "Config"=w140) -> ("Error Out"=w149:errorcluster)  [unwired: 8 in, 1 out]
              }
            }
          }
          frame "Write config" {
            n57 = Variant To Data(error in=w156, type=T1 {"DAQ"={"Data"={"Live"={"t0"=timestamp(0 s since 1904-01-01), "dt"=1.0, "Y"=[]}, "Accumulated"={"t0"=timestamp(0 s since 1904-01-01), "dt"=1.0, "Y"=[]}, "Averaged"={"t0"=timestamp(0 s since 1904-01-01), "dt"=1.0, "Y"=[]}, "data array"=[], "live time array"=[], "Live (decimated)"={"t0"=timestamp(0 s since 1904-01-01), "dt"=1.0, "Y"=[]}}, "Config"={"Input Config"=0, "Card"=enum."USB-6211", "100% Reflectance Standard (V)"=0.0, "Input Channel"="", "Average number of points"=0.0, "Trigger Level (V)"=0.0, "Rate (Hz)"=0, "End Time (s)"=0.0}, "Indicators"={"Final number of points"=0.0, "Number of samples"=0.0, "dt"=0.0, "Shots"=0, "Shot counter"=0, "Test counter"=0, "Background level (V)"=0.0, "DAQ task"="", "timestamp of data"=timestamp(0 s since 1904-01-01), "Test Type"=enum."A-Test"}}, "Shutter"={"Open command string"="", "VISA"={"Timeout (ms)"=0, "Resource Name"="", "Baud Rate"=0, "Data Bits"=0, "Parity"=0, "Stop Bits"=0, "Flow Control"=0}}, "Monochromator"={"Type"=enum."Oriel", "Wavelength (nm)"=0.0, "Grating, gr/mm"=enum."2400", "Grating mode"=enum."Unknown", "Spectrum mode"={"Spectrum mode?"=FALSE, "Start wavelength (nm)"=0.0, "End wavelength (nm)"=0.0, "Wavelength step (nm)"=0.0, "Wavelength array"=[], "array index"=0}, "PTI"={"Delay before read (ms)"=0, "Mono 1"={"Timeout (ms)"=0, "Resource Name"="", "Baud Rate"=0, "Data Bits"=0, "Parity"=0, "Stop Bits"=0, "Flow Control"=0}, "Mono 2"={"Timeout (ms)"=0, "Resource Name"="", "Baud Rate"=0, "Data Bits"=0, "Parity"=0, "Stop Bits"=0, "Flow Control"=0}, "Two PTI Monochromators?"=FALSE}, "Oriel (custom)"={"reference"=refnum}, "Force wavelength confirmation (PTI)?"=FALSE}, "Test"={"Config"={"Amplification Factor"=0.0, "100% Reflectance Standard"=0.0, "Calculation Method"=enum."Reflectance", "Option to discard new data?"=FALSE, "Mode"=enum."Spectrum", "Number of Averages"=0, "B Test?"=FALSE}, "Indicators"={"DAQ Background Level (V)"=2.0, "A-Test Counter"=2, "B-Test Counter"=2, "Type"=enum."A-Test", "Scope Background Level (Amps)"=2.0, "TAS only?"=FALSE}}, "Scope"={"Config"={"VISA Resource"="", "Model"=enum."DPO 3012", "Timebase"=0.0, "Timeout (ms)"=0, "TAS"={"Vertical Range (V)"=0.0, "Vertical Offset (0.0 divs)"=0.0, "Bandwidth"=0, "Probe Attenuation (10.0)"=0.0, "Vertical Coupling"=0, "Impedance"=0, "Multiplication factor"=0.0, "Channel"=enum."Channel 1"}, "TPC"={"Vertical Range (V)"=0.0, "Vertical Offset (0.0 divs)"=0.0, "Bandwidth"=0, "Probe Attenuation (10.0)"=0.0, "Vertical Coupling"=0, "Impedance"=0, "Multiplication factor"=0.0, "Channel"=enum."Channel 1"}, "Trigger"={"Mode"=enum."Laser (TAS)", "Source "=enum."Channel 1", "PIA"={"Test LEDs"=FALSE, "LED line"="", "LED off (s)"=0.0, "LED on (s)"=0.0}, "Threshold (V)"=0.0004}}, "Indicators"={"Setup"={"Final number of points"=0.0, "Pretrigger points"=0.0, "Number of readouts"=0, "Model"={"Acquisition Type"=0, "Record length (points)"=0, "Averages on scope"=0, "Average number of points"=0.0}}, "Timestamp of Data"=timestamp(0 s since 1904-01-01)}, "Data"={"TPC"={"Live data"={"t0"=timestamp(0 s since 1904-01-01), "dt"=1.0, "Y"=[]}, "Averaged data"={"t0"=timestamp(0 s since 1904-01-01), "dt"=1.0, "Y"=[]}, "Accumulated data"={"t0"=timestamp(0 s since 1904-01-01), "dt"=1.0, "Y"=[]}, "Final data"={"t0"=timestamp(0 s since 1904-01-01), "dt"=1.0, "Y"=[]}}, "TAS"={"Live data"={"t0"=timestamp(0 s since 1904-01-01), "dt"=1.0, "Y"=[]}, "Averaged data"={"t0"=timestamp(0 s since 1904-01-01), "dt"=1.0, "Y"=[]}, "Accumulated data"={"t0"=timestamp(0 s since 1904-01-01), "dt"=1.0, "Y"=[]}, "Final data"={"t0"=timestamp(0 s since 1904-01-01), "dt"=1.0, "Y"=[]}}, "Time arrays"={"Time array (decimated)"=[], "waveform"={"t0"=timestamp(0 s since 1904-01-01), "dt"=1.0, "Y"=[]}}}, "Test"={"Config"={"Amplification Factor"=2.0, "100% Reflectance Standard"=2.0, "Calculation Method"=enum."Reflectance", "Option to discard new data?"=FALSE, "Mode"=enum."Spectrum", "Number of Averages"=0, "B Test?"=FALSE}, "Indicators"={"DAQ Background Level (V)"=2.0, "A-Test Counter"=2, "B-Test Counter"=2, "Type"=enum."A-Test", "Scope Background Level (Amps)"=2.0, "TAS only?"=FALSE}}}, "Colour wheel"={"Reference"=0, "Colour Wheel Wavelengths"=[], "Waveform Index"=0, "COM Port"="", "Enabled?"=FALSE}, "File IO"={"Output Folder"=path "", "Error file"=path "", "Config file"=path "", "File prefix"="", "Waveform read"={"t0"=timestamp(0 s since 1904-01-01), "dt"=1.0, "Y"=[]}}} ("Parameters"), Variant=w158) -> (data=w150:T1, error out=w155:errorcluster)
            n58 = Unbundle By Name(w150) -> ("File IO.Config file"=w154:path)
            n59 = call-poly <userlib>:"Valid Path__ogtk.vi"("path"=w154) -> ("valid"=w159:bool)
            n60 = case shown="True" w159 {
              tunnel: [w162 w166] -> w160
              tunnel: w155 -> [w162 w171]
              tunnel: w154 -> [_ w173]
              tunnel: w150 -> [_ w164]
              tunnel: [w161 w165] -> w153
              tunnel: w151 -> [w161 w165]
              frame False {
              }
              frame True {
                n61 = call <vilib>:"Open Config Data.vi"("error in (no error)"=w171, "configuration file path"=w173) -> ("error out"=w170:errorcluster, "refnum"=w172:T38)  [unwired: 7 in, 1 out]
                n62 = call "System Cluster to Config Cluster Conversion.vi"("System Cluster"=w164) -> ("Config Cluster"=w163:T37)  [unwired: 9 in, 1 out]
                n63 = call <userlib>:"Write INI Cluster__ogtk.vi"("error in (no error)"=w170, "INI Fomatted Cluster"=w163, "refnum"=w172) -> ("error out"=w169:errorcluster, "dup refnum"=w168:T38)  [unwired: 7 in]
                n64 = call <vilib>:"Close Config Data.vi"("error in (no error)"=w169, "refnum"=w168) -> ("error out"=w167:errorcluster)  [unwired: 8 in, 1 out]
                n65 = call "Set all config data API.vi"("Error In"=w167, "Config"=w164) -> ("Error Out"=w166:errorcluster)  [unwired: 8 in, 1 out]
              }
            }
          }
          frame "Save parameters" {
            n66 = Variant To Data(error in=w178, type=T1 {"DAQ"={"Data"={"Live"={"t0"=timestamp(0 s since 1904-01-01), "dt"=1.0, "Y"=[]}, "Accumulated"={"t0"=timestamp(0 s since 1904-01-01), "dt"=1.0, "Y"=[]}, "Averaged"={"t0"=timestamp(0 s since 1904-01-01), "dt"=1.0, "Y"=[]}, "data array"=[], "live time array"=[], "Live (decimated)"={"t0"=timestamp(0 s since 1904-01-01), "dt"=1.0, "Y"=[]}}, "Config"={"Input Config"=10106, "Card"=enum."USB-6211", "100% Reflectance Standard (V)"=1.0, "Input Channel"="Dev2/ai0", "Average number of points"=50.0, "Trigger Level (V)"=0.4, "Rate (Hz)"=250000, "End Time (s)"=1.0}, "Indicators"={"Final number of points"=0.0, "Number of samples"=0.0, "dt"=0.0, "Shots"=1, "Shot counter"=0, "Test counter"=0, "Background level (V)"=0.0, "DAQ task"="", "timestamp of data"=timestamp(0 s since 1904-01-01), "Test Type"=enum."A-Test"}}, "Shutter"={"Open command string"="", "VISA"={"Timeout (ms)"=0, "Resource Name"="", "Baud Rate"=0, "Data Bits"=0, "Parity"=0, "Stop Bits"=0, "Flow Control"=0}}, "Monochromator"={"Type"=enum."Oriel", "Wavelength (nm)"=0.0, "Grating, gr/mm"=enum."2400", "Grating mode"=enum."Unknown", "Spectrum mode"={"Spectrum mode?"=FALSE, "Start wavelength (nm)"=0.0, "End wavelength (nm)"=0.0, "Wavelength step (nm)"=0.0, "Wavelength array"=[], "array index"=0}, "PTI"={"Delay before read (ms)"=0, "Mono 1"={"Timeout (ms)"=0, "Resource Name"="", "Baud Rate"=0, "Data Bits"=0, "Parity"=0, "Stop Bits"=0, "Flow Control"=0}, "Mono 2"={"Timeout (ms)"=0, "Resource Name"="", "Baud Rate"=0, "Data Bits"=0, "Parity"=0, "Stop Bits"=0, "Flow Control"=0}, "Two PTI Monochromators?"=FALSE}, "Oriel (custom)"={"reference"=refnum}, "Force wavelength confirmation (PTI)?"=FALSE}, "Test"={"Config"={"Amplification Factor"=0.0, "100% Reflectance Standard"=0.0, "Calculation Method"=enum."Reflectance", "Option to discard new data?"=FALSE, "Mode"=enum."Spectrum", "Number of Averages"=0, "B Test?"=FALSE}, "Indicators"={"DAQ Background Level (V)"=0.0, "A-Test Counter"=0, "B-Test Counter"=0, "Type"=enum."A-Test", "Scope Background Level (Amps)"=2.0, "TAS only?"=FALSE}}, "Scope"={"Config"={"VISA Resource"="USB0::0x0699::0x039D::C010764::INSTR", "Model"=enum."DPO 2012B", "Timebase"=0.0004, "Timeout (ms)"=60000, "TAS"={"Vertical Range (V)"=2.0, "Vertical Offset (0.0 divs)"=0.0, "Bandwidth"=0, "Probe Attenuation (10.0)"=1.0, "Vertical Coupling"=1, "Impedance"=0, "Multiplication factor"=1.0, "Channel"=enum."Channel 1"}, "TPC"={"Vertical Range (V)"=2.0, "Vertical Offset (0.0 divs)"=0.0, "Bandwidth"=0, "Probe Attenuation (10.0)"=1.0, "Vertical Coupling"=1, "Impedance"=0, "Multiplication factor"=1.0, "Channel"=enum."None"}, "Trigger"={"Mode"=enum."Laser (TAS)", "Source "=enum."Aux", "PIA"={"Test LEDs"=FALSE, "LED line"="", "LED off (s)"=0.0, "LED on (s)"=0.0}, "Threshold (V)"=0.8}}, "Indicators"={"Setup"={"Final number of points"=0.0, "Pretrigger points"=0.0, "Number of readouts"=0, "Model"={"Acquisition Type"=4, "Record length (points)"=1000, "Averages on scope"=4, "Average number of points"=10.0}}, "Timestamp of Data"=timestamp(0 s since 1904-01-01)}, "Data"={"TPC"={"Live data"={"t0"=timestamp(0 s since 1904-01-01), "dt"=1.0, "Y"=[]}, "Averaged data"={"t0"=timestamp(0 s since 1904-01-01), "dt"=1.0, "Y"=[]}, "Accumulated data"={"t0"=timestamp(0 s since 1904-01-01), "dt"=1.0, "Y"=[]}, "Final data"={"t0"=timestamp(0 s since 1904-01-01), "dt"=1.0, "Y"=[]}}, "TAS"={"Live data"={"t0"=timestamp(0 s since 1904-01-01), "dt"=1.0, "Y"=[]}, "Averaged data"={"t0"=timestamp(0 s since 1904-01-01), "dt"=1.0, "Y"=[]}, "Accumulated data"={"t0"=timestamp(0 s since 1904-01-01), "dt"=1.0, "Y"=[]}, "Final data"={"t0"=timestamp(0 s since 1904-01-01), "dt"=1.0, "Y"=[]}}, "Time arrays"={"Time array (decimated)"=[], "waveform"={"t0"=timestamp(0 s since 1904-01-01), "dt"=1.0, "Y"=[]}}}, "Test"={"Config"={"Amplification Factor"=0.0, "100% Reflectance Standard"=0.0, "Calculation Method"=enum."Reflectance", "Option to discard new data?"=FALSE, "Mode"=enum."Spectrum", "Number of Averages"=100, "B Test?"=FALSE}, "Indicators"={"DAQ Background Level (V)"=2.0, "A-Test Counter"=2, "B-Test Counter"=2, "Type"=enum."A-Test", "Scope Background Level (Amps)"=2.0, "TAS only?"=FALSE}}}, "Colour wheel"={"Reference"=0, "Colour Wheel Wavelengths"=[], "Waveform Index"=0, "COM Port"="", "Enabled?"=FALSE}, "File IO"={"Output Folder"=path "C:/Users/Abigail/Documents/Imperial Optical software/Optical Software Code Simplified/Output", "Error file"=path "C:/Users/Abigail/Documents/Imperial Optical software/Optical Software Code Simplified/Error Log.txt", "Config file"=path "C:/Users/Abigail/Documents/Imperial Optical software/Optical Software Code Simplified/Config.ini", "File prefix"="", "Waveform read"={"t0"=timestamp(0 s since 1904-01-01), "dt"=1.0, "Y"=[]}}} ("Config 2"), Variant=w179) -> (data=w174:T1, error out=w176:errorcluster)
            n67 = call "Save parameters to file.vi"("error in"=w176, "Config"=w174) -> ("error out"=w175:errorcluster)  [unwired: 9 in]
          }
          frame "Update file prefix" {
            n68 = Variant To Data(error in=w187, type="", Variant=w188) -> (data=w184:string, error out=w186:errorcluster)
            n69 = Bundle By Name(cluster=w183, "File prefix"=w184) -> (w182:T29)
          }
        }
      }
      event Value Change {
        n70 = event-data() -> ("NewVal"=w193:T30)  [unwired: 1 in]
        n71 = case shown="\"Update file prefix\"" w193 {
          tunnel: [w197 w201 w205 w209 w213 w221 w225 w227 w231 w233 w235] -> w195
          tunnel: w194 -> [w198 w202 w206 w210 _ w222 w226 w228 w231 w233 w235]
          tunnel: w192 -> [w196 w203 w207 w211 w214 w220 w223 w229 w230 w232 w234]
          tunnel: [w196 w203 w207 w211 w214 w220 w223 w229 w230 w232 w234] -> w191
          tunnel: "Config" -> [_ _ _ _ _ _ w224 _ _ _ _]
          frame "Start" {
            n72 = call "Start API.vi"("File IO parameters"=w196, "Error In"=w198) -> ("Error Out"=w197:errorcluster)  [unwired: 9 in]
          }
          frame "Write waveform" {
            w199 = dbl[][] []  # Waveform Data
            n73 = call "Write waveform API.vi"("Error In"=w202, "Waveform name"="Test", "Waveform Data"=w199) -> ("Error Out"=w201:errorcluster)  [unwired: 8 in]
          }
          frame "Read waveform" {
            n74 = call "Read waveform API.vi"("Error In"=w206, "Waveform name"="Test") -> ("Error Out"=w205:errorcluster)  [unwired: 9 in]
          }
          frame "Send waveform to processing" {
            n75 = call "Send waveform API.vi"("Error In"=w210, "Waveform name"="Test waveform") -> ("Error Out"=w209:errorcluster)  [unwired: 9 in]
          }
          frame "Log error" {
            n76 = xnode "Error Ring"() -> ("error out"=w212:errorcluster)
            n77 = call "Log error API.vi"("Error In"=w212) -> ("Error Out"=w213:errorcluster)  [unwired: 10 in]
          }
          frame "Stop" {
            n78 = call "Stop API.vi"("Error In"=w222) -> ("Error Out"=w221:errorcluster)  [unwired: 10 in]
          }
          frame "Write config" {
            n79 = call "Write config API.vi"("System parameters"=w224, "Error In"=w226) -> ("Error Out"=w225:errorcluster)  [unwired: 9 in]
          }
          frame "Read config" {
            n80 = call "Read config API.vi"("Error In"=w228) -> ("Error Out"=w227:errorcluster)  [unwired: 10 in]
          }
          frame "Save parameters" {
          }
          frame "Delete waveform" {
          }
          frame "Update file prefix" {
          }
        }
      }
      event User Event {
        n81 = event-data() -> ("Error Cluster"=w237:errorcluster)  [unwired: 1 in]
        n82 = call "Log error API.vi"("Error In"=w237) -> ("Error Out"=w236:errorcluster)  [unwired: 10 in]
      }
    }
  }
  "Error Out" <- w11
  n83 = Unregister For Events(event registration refnum=w13) -> ()  [unwired: 1 in, 1 out]
